vi "timeStamp_compare.vi"(8 "TIME STRING 2":string, 9 "TIME STRING 1":string, 11 "TIME FORMAT":u16(ring) items=["MMM DD, YYYY", "YYMMDDhhmmss", "DD/MM/YY", "HH:MM:SS", "MMM DD, YYYY | hh:mm:ss"]) -> (0 "SUCCESS?":bool, 3 "RESULT":i32)   [LabVIEW 2018, in "db_lib R3.lvlib"]
uses:
  db_lib R3.lvlib
panel:
  # "STR1 > STR2 : RESULT IS 1\nSTR1 < STR2 : RESULT IS -1\nSTR1 = STR2 : RESULT IS 0"
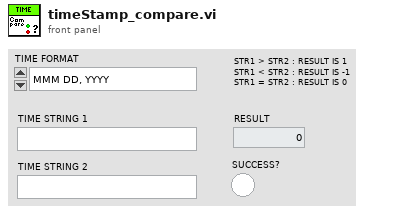
[diagram p1: front panel]
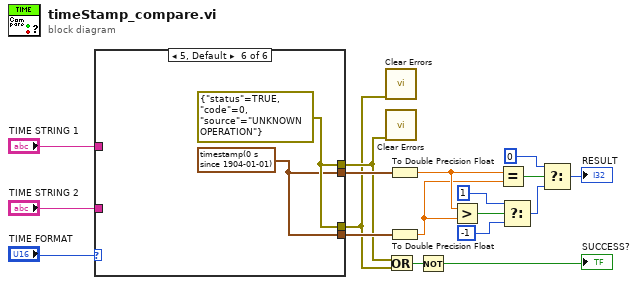
[diagram p0: block diagram]
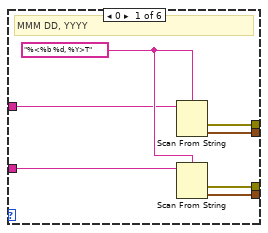
[diagram p2: hidden frame]
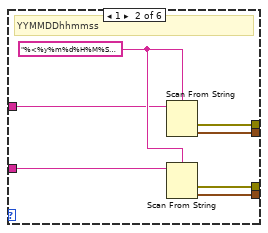
[diagram p3: hidden frame]
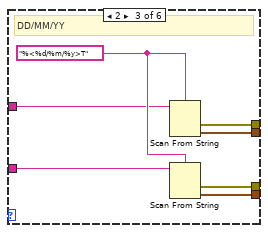
[diagram p4: hidden frame]
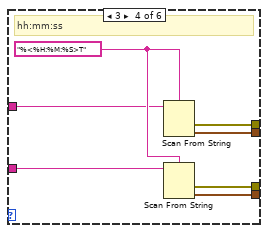
[diagram p5: hidden frame]
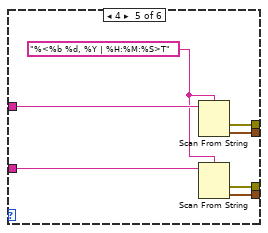
[diagram p6: hidden frame]
diagram:
  n1 = case shown="5, Default" "TIME FORMAT" {
    tunnel: [w25 w32 w39 w46 w52 w54] -> w13
    tunnel: [w24 w31 w38 w45 w53 w55] -> w3
    tunnel: "TIME STRING 1" -> [w19 w26 w34 w43 w51 _]
    tunnel: "TIME STRING 2" -> [w20 w27 w33 w42 w49 _]
    tunnel: [w22 w28 w36 w41 w48 w55] -> w2
    tunnel: [w21 w29 w35 w40 w47 w54] -> w12
    frame 0 {
      w23 = "%<%b %d, %Y>T" ("format string")
      # "MMM DD, YYYY"
      n2 = Scan From String(format string=w23, input string=w19) -> (error out=w24:errorcluster, output 1=w25:timestamp)  [unwired: 3 in, 2 out]
      n3 = Scan From String(format string=w23, input string=w20) -> (error out=w22:errorcluster, output 1=w21:timestamp)  [unwired: 3 in, 2 out]
    }
    frame 1 {
      w30 = "%<%y%m%d%H%M%S>T" ("format string")
      # "YYMMDDhhmmss"
      n4 = Scan From String(format string=w30, input string=w26) -> (error out=w31:errorcluster, output 1=w32:timestamp)  [unwired: 3 in, 2 out]
      n5 = Scan From String(format string=w30, input string=w27) -> (error out=w28:errorcluster, output 1=w29:timestamp)  [unwired: 3 in, 2 out]
    }
    frame 2 {
      w37 = "%<%d/%m/%y>T" ("format string")
      # "DD/MM/YY"
      n6 = Scan From String(format string=w37, input string=w34) -> (error out=w38:errorcluster, output 1=w39:timestamp)  [unwired: 3 in, 2 out]
      n7 = Scan From String(format string=w37, input string=w33) -> (error out=w36:errorcluster, output 1=w35:timestamp)  [unwired: 3 in, 2 out]
    }
    frame 3 {
      w44 = "%<%H:%M:%S>T" ("format string")
      # "hh:mm:ss"
      n8 = Scan From String(format string=w44, input string=w43) -> (error out=w45:errorcluster, output 1=w46:timestamp)  [unwired: 3 in, 2 out]
      n9 = Scan From String(format string=w44, input string=w42) -> (error out=w41:errorcluster, output 1=w40:timestamp)  [unwired: 3 in, 2 out]
    }
    frame 4 {
      w50 = "%<%b %d, %Y | %H:%M:%S>T" ("format string")
      n10 = Scan From String(format string=w50, input string=w51) -> (error out=w53:errorcluster, output 1=w52:timestamp)  [unwired: 3 in, 2 out]
      n11 = Scan From String(format string=w50, input string=w49) -> (error out=w48:errorcluster, output 1=w47:timestamp)  [unwired: 3 in, 2 out]
    }
    frame 5, Default {
      w55 = errorcluster {"status"=TRUE, "code"=0, "source"="UNKNOWN OPERATION"} ("error IO")
      w54 = timestamp(0 s since 1904-01-01)
    }
  }
  n12 = call <vilib>:"Clear Errors.vi"("error in (no error)"=w2) -> ()  [unwired: 5 in, 2 out]
  n13 = call <vilib>:"Clear Errors.vi"("error in (no error)"=w3) -> ()  [unwired: 5 in, 2 out]
  n14 = Or(x=w3, y=w2) -> (x .or. y?=w15:bool)
  n15 = To Double Precision Float(number=w13) -> (double precision float=w9:dbl)
  n16 = To Double Precision Float(number=w12) -> (double precision float=w1:dbl)
  n17 = Not(x=w15) -> (.not. x?=→"SUCCESS?":bool)
  n18 = Greater?(x=w9, y=w1) -> (0:w8:bool)
  n19 = Equal?(x=w9, y=w1) -> (x = y?=w11:bool)
  n20 = Select(t=1, s=w8, f=-1) -> (s? t:f=w5:i32)
  n21 = Select(t=0, s=w11, f=w5) -> (s? t:f=→"RESULT":i32)
